vi "read_n_raw_records.vi"(8 "error in":errorcluster, 10 "Num records":i32, 11 "Byte Stream File in":refnum<file>) -> (0 "error out":errorcluster, 1 "Input data":waveform(dbl)[][][](array[waveform]), 2 "Timestamps":timestamp[][](array[timestamp]), 3 "Byte Stream File out":refnum<file>)   [LabVIEW 2024]
panel:
  # "Read this many records, or all if 0"
  # "Read multiple raw data records"
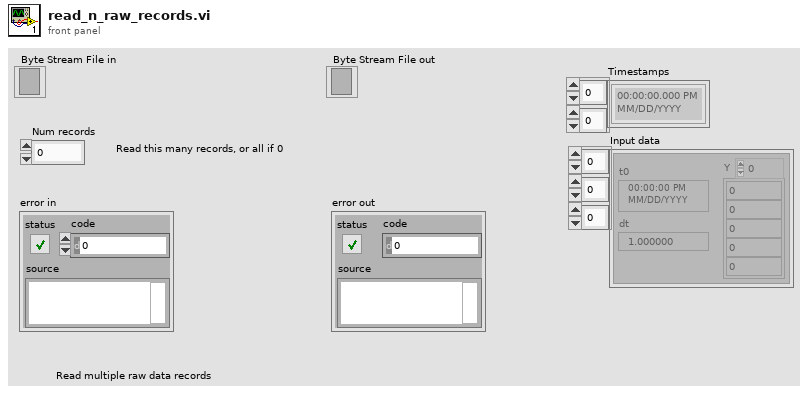
[diagram p1: front panel]
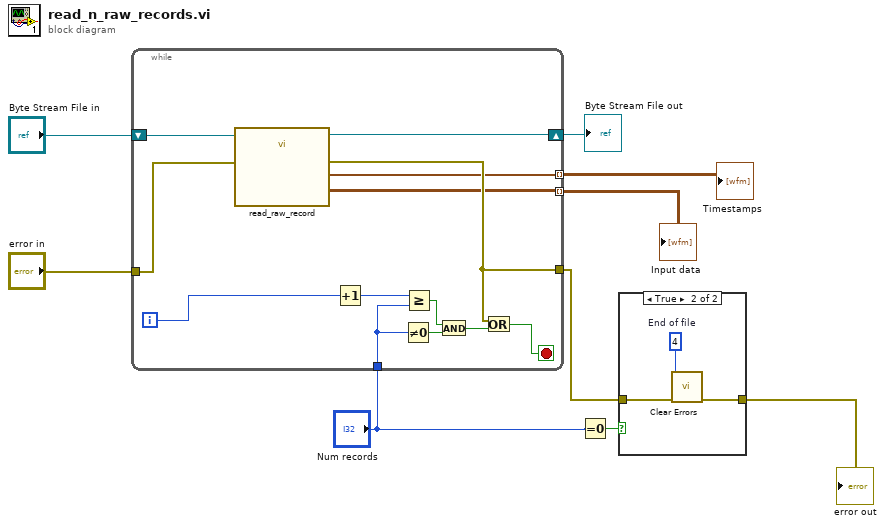
[diagram p0: block diagram]
diagram:
  n1 = while {
    tunnel: "Num records" -> [w20]
    tunnel: "error in" -> [w19]
    tunnel: [w16] -> w2
    tunnel: [w13] -> w6 mode=indexing
    tunnel: [w12] -> w5 mode=indexing
    shift-right: [w17] -> w7
    shift-left: "Byte Stream File in" -> [w18]
    i -> [w11]
    stop <- w14 stop-if-true
    n2 = call "read_raw_record.vi"("error in"=w19, "Byte Stream File in"=w18) -> ("error out"=w16:errorcluster, "Input data"=w12:waveform(dbl)[][], "Timestamps"=w13:timestamp[], "Byte Stream File out"=w17:refnum<file>)  [unwired: 6 in]
    n3 = Increment(x=w11) -> (x+1=w10:i32)
    n4 = Not Equal To 0?(x=w20) -> (x != 0?=w22:bool)
    n5 = Greater Or Equal?(x=w10, y=w20) -> (x >= y?=w21:bool)
    n6 = And(x=w21, y=w22) -> (x .and. y?=w15:bool)
    n7 = Or(x=w16, y=w15) -> (x .or. y?=w14:bool)
  }
  "Byte Stream File out" <- w7
  "Timestamps" <- w6
  "Input data" <- w5
  n8 = Equal To 0?(x="Num records") -> (x = 0?=w3:bool)
  n9 = case shown="True" w3 {
    tunnel: w2 -> [w23 w25]
    tunnel: [w23 w24] -> w1
    frame False {
    }
    frame True {
      w26 = 4  # End of file
      n10 = call <vilib>:"Clear Errors.vi"("error in (no error)"=w25, "specific error code to clear (0: all)"=w26) -> ("error out"=w24:errorcluster)  [unwired: 4 in, 1 out]
    }
  }
  "error out" <- w1
